vi "Open Lift.vi"   [LabVIEW 2014]
uses:
  <vilib>/Rock Robotics/WPI/CAN/TalonSRX/WPI_CANTalonSRX_APIControlMode.ctl
  Robot Global Data.vi
  <vilib>/Rock Robotics/WPI/MotorControl/WPI_MotorControlOpenCANTalonSRX.vi
  <vilib>/Rock Robotics/WPI/Solenoid/WPI_SolenoidOpenSingle.vi
  <vilib>/Rock Robotics/WPI/Solenoid/WPI_SolenoidOpenDouble.vi
types:
  T1 = typedef "WPI_CANTalonSRX_APIControlMode.ctl" = enum8{"Percent VBus", "Speed", "Position", "Slave", "Unchanged / Invalid"}
  T2 = typedef "FPGA_DIOChannel.ctl" = enum8{"DIO 0", "DIO 1", "DIO 2", "DIO 3", "DIO 4", "DIO 5", "DIO 6", "DIO 7", "DIO 8", "DIO 9", "DIO MXP 0", "DIO MXP 1", "DIO MXP 2", "DIO MXP 3", "DIO MXP 4", "DIO MXP 5", "DIO MXP 6", "DIO MXP 7", "DIO MXP 8", "DIO MXP 9", "DIO MXP 10", "DIO MXP 11", "DIO MXP 12", "DIO MXP 13", "DIO MXP 14", "DIO MXP 15", "Invalid"}
  T3 = cluster{"Lift Motors":cluster{"Left Lift":dbl, "Right Lift":dbl}, "Sensors":cluster{"Limit Switches":cluster{"Bottom IR":T2, "Top IR":T2}, "Encoders":cluster{"Lift Encoder A Pin":T2, "Lift Encoder B Pin":T2}}, "Solenoids":cluster{"Left Clamp FWD":dbl, "Right Clamp FWD":dbl, "Brake":dbl, "Left Clamp BCK":dbl, "Right Clamp BCK":dbl, "Left Clamp PModule":dbl, "Right Clamp PModule":dbl, "Brake PModule":dbl}, "Drive Motors":cluster{"Rear Left Motor":dbl, "Rear Right Motor":dbl, "Front Left Motor":dbl, "Front Right Motor":dbl}}
  T4 = typedef "WPI_SolenoidDevRef.ctl" = cluster{"DevStatus":errorcluster, "Pneumatics Control Module":u8, "Forward Solenoid Channel":T5, "Reverse Solenoid Channel":T5}
  T5 = typedef "WPI_SolenoidChannel.ctl" = enum8{"Solenoid 0", "Solenoid 1", "Solenoid 2", "Solenoid 3", "Solenoid 4", "Solenoid 5", "Solenoid 6", "Solenoid 7", "Invalid"}
  T6 = typedef "WPI_MotorControlDeviceRef.ctl" = cluster{"DeviceStatus":errorcluster, "Type":T7, "PWM":cluster{"Controller":T8, "PWM Channel":T9, "DeadBand":T10}, "CAN":cluster{"Device Number":u8, "Control Mode":T11, "Semaphore":T12, "Max Vout":dbl, "TalonSRX Control Mode":T1}, "Invert":bool, "TransformRef":T13, "InvTransformRef":T13}
  T7 = typedef "WPI_MotorControlType.ctl" = enum16{"PWM", "CAN", "CANTalonSRX"}
  T8 = typedef "FPGA_TypedefDigitalModule.ctl" = enum16{"Controller 1"}
  T9 = typedef "FPGA_DIOPWMChannel.ctl" = enum8{"PWM 0", "PWM 1", "PWM 2", "PWM 3", "PWM 4", "PWM 5", "PWM 6", "PWM 7", "PWM 8", "PWM 9", "PWM MXP 0", "PWM MXP 1", "PWM MXP 2", "PWM MXP 3", "PWM MXP 4", "PWM MXP 5", "PWM MXP 6", "PWM MXP 7", "PWM MXP 8", "PWM MXP 9", "Invalid"}
  T10 = typedef "WPI_PWMDeadband.ctl" = cluster{"Name":string, "maxPositivePwm":i32, "minPositivePwm":i32, "centerPwm":i32, "maxNegativePwm":i32, "minNegativePwm":i32, "angularRange":u16}
  T11 = typedef "WPI_CANJaguar_ControlMode.ctl" = enum8{"Percent VBus", "Current", "Speed", "Position", "Voltage"}
  T12 = typedef "Semaphore RefNum" = refnum<k1>
  T13 = typedef "WPI_PWMTransform_ConPane.ctl" = refnum<vi>
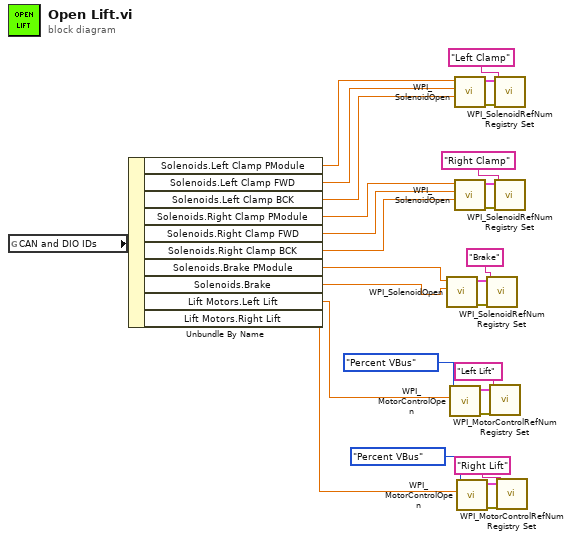
[diagram p0: block diagram]
diagram:
  n1 = global read "Robot Global Data.vi" "CAN and DIO IDs"() -> (w11:T3)
  n2 = Unbundle By Name(w11) -> ("Solenoids.Left Clamp PModule"=w1:dbl, "Solenoids.Left Clamp FWD"=w2:dbl, "Solenoids.Left Clamp BCK"=w3:dbl, "Solenoids.Right Clamp PModule"=w4:dbl, "Solenoids.Right Clamp FWD"=w5:dbl, "Solenoids.Right Clamp BCK"=w6:dbl, "Solenoids.Brake PModule"=w7:dbl, "Solenoids.Brake"=w8:dbl, "Lift Motors.Left Lift"=w10:dbl, "Lift Motors.Right Lift"=w9:dbl)
  n3 = call-poly <vilib>:"WPI_SolenoidOpen.vi"("Solenoid Channel"=w8, "Pneumatics Control Module (0)"=w7) -> ("error out"=w28:errorcluster, "SolenoidDevRef"=w27:T4)  [unwired: 8 in]
  n4 = call-poly <vilib>:"WPI_MotorControlOpen.vi"("Device Number"=w10, "Control Mode"=WPI_CANTalonSRX_APIControlMode."Percent VBus") -> ("error out"=w25:errorcluster, "MotorControlDeviceRef"=w17:T6)  [unwired: 8 in]
  n5 = call-poly <vilib>:"WPI_SolenoidOpen.vi"("Reverse Solenoid Channel"=w3, "Forward Solenoid Channel"=w2, "Pneumatics Control Module (0)"=w1) -> ("error out"=w14:errorcluster, "SolenoidDevRef"=w13:T4)  [unwired: 7 in]
  n6 = call-poly <vilib>:"WPI_SolenoidOpen.vi"("Reverse Solenoid Channel"=w6, "Forward Solenoid Channel"=w5, "Pneumatics Control Module (0)"=w4) -> ("error out"=w20:errorcluster, "SolenoidDevRef"=w19:T4)  [unwired: 7 in]
  n7 = call-poly <vilib>:"WPI_MotorControlOpen.vi"("Device Number"=w9, "Control Mode"=WPI_CANTalonSRX_APIControlMode."Percent VBus") -> ("error out"=w21:errorcluster, "MotorControlDeviceRef"=w16:T6)  [unwired: 8 in]
  n8 = call <vilib>:"WPI_SolenoidRefNum Registry Set.vi"("error in (no error)"=w28, "refnum name"="Brake", "SolenoidDevRef"=w27) -> ()  [unwired: 7 in, 2 out]
  n9 = call <vilib>:"WPI_MotorControlRefNum Registry Set.vi"("error in (no error)"=w25, "refnum name"="Left Lift", "MotorControlDevRef"=w17) -> ()  [unwired: 7 in, 2 out]
  n10 = call <vilib>:"WPI_SolenoidRefNum Registry Set.vi"("error in (no error)"=w14, "refnum name"="Left Clamp", "SolenoidDevRef"=w13) -> ()  [unwired: 7 in, 2 out]
  n11 = call <vilib>:"WPI_SolenoidRefNum Registry Set.vi"("error in (no error)"=w20, "refnum name"="Right Clamp", "SolenoidDevRef"=w19) -> ()  [unwired: 7 in, 2 out]
  n12 = call <vilib>:"WPI_MotorControlRefNum Registry Set.vi"("error in (no error)"=w21, "refnum name"="Right Lift", "MotorControlDevRef"=w16) -> ()  [unwired: 7 in, 2 out]
